vi "Close.vi"(8 "error in (no error)":errorcluster, 11 "Logger Level in":refnum<class "Logger Level.lvclass">) -> (0 "error out":errorcluster, 3 "Logger Level out":refnum<class "Logger Level.lvclass">)   [LabVIEW 2020, in "Logger Level.lvlib" / "Logger Level.lvclass"]
uses:
  Logger Level.lvclass
  <vilib>/ActorFramework/Stop Msg/Stop Msg.lvclass
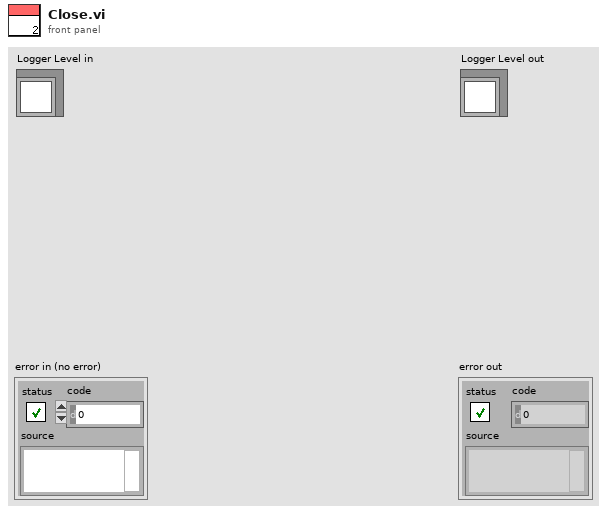
[diagram p1: front panel]
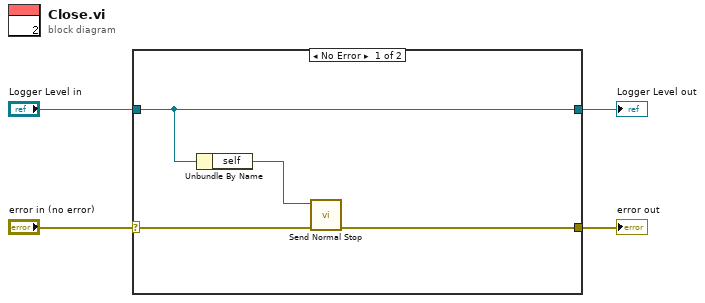
[diagram p0: block diagram]
diagram:
  n1 = case shown="No Error" "error in (no error)" {
    selector: "error in (no error)" -> [w7 w10]
    tunnel: "Logger Level in" -> [w8 w9]
    tunnel: [w6 w10] -> w1
    tunnel: [w8 w9] -> w2
    frame No Error {
      n2 = Unbundle By Name(w8) -> ("self"=w5:refnum<class "Message Enqueuer.lvclass">)
      n3 = call <vilib>:"Send Normal Stop.vi"("error in (no error)"=w7, "Message Enqueuer"=w5) -> ("error out"=w6:errorcluster)  [unwired: 9 in]
    }
    frame Error {
    }
  }
  "error out" <- w1
  "Logger Level out" <- w2
